vi "Initialize.vi"(8 "error in (no error)":errorcluster, 10 "Interval (ms)":dbl, 11 "Gate in":refnum<class "Gate.lvclass">) -> (0 "error out":errorcluster, 3 "Gate out":refnum<class "Gate.lvclass">)   [LabVIEW 2015, in "Gate.lvclass"]
uses:
  Gate.lvclass
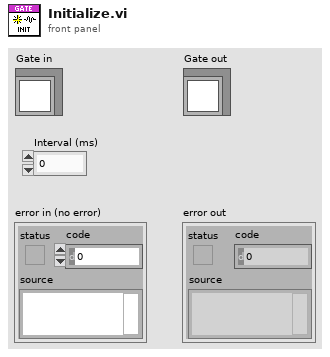
[diagram p1: front panel]
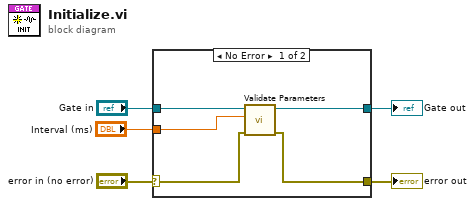
[diagram p0: block diagram]
diagram:
  n1 = case shown="No Error" "error in (no error)" {
    selector: "error in (no error)" -> [w8 w12]
    tunnel: [w7 w12] -> w4
    tunnel: [w9 w11] -> w2
    tunnel: "Gate in" -> [w10 w11]
    tunnel: "Interval (ms)" -> [w6 _]
    frame No Error {
      n2 = call "Validate Parameters.vi"("error in (no error)"=w8, "Interval (ms)"=w6, "Gate in"=w10) -> ("error out"=w7:errorcluster, "Gate out"=w9:refnum<class "Gate.lvclass">)  [unwired: 7 in]
    }
    frame Error {
    }
  }
  "error out" <- w4
  "Gate out" <- w2
